vi "时间波形函数.vi"() -> ()   [LabVIEW 2023]
panel:
  out "Waveform Chart":waveform(dbl)[](graph)
  out "Waveform Graph 2":waveform(dbl)[](graph)
  out "appended array":waveform(dbl)[](array[waveform])
  out "Waveform Graph":waveform(dbl)(graph)
  out "output waveform":waveform(dbl)
  # "时间波形函数"
  # "t0（采样起始时间）、dt（采样间隔时间）、Y（数据，一维数组表示的每个点对应 Y 轴上的值）、attributes（波形的一些属性）"
  # "设置 和 读取 波形属性"
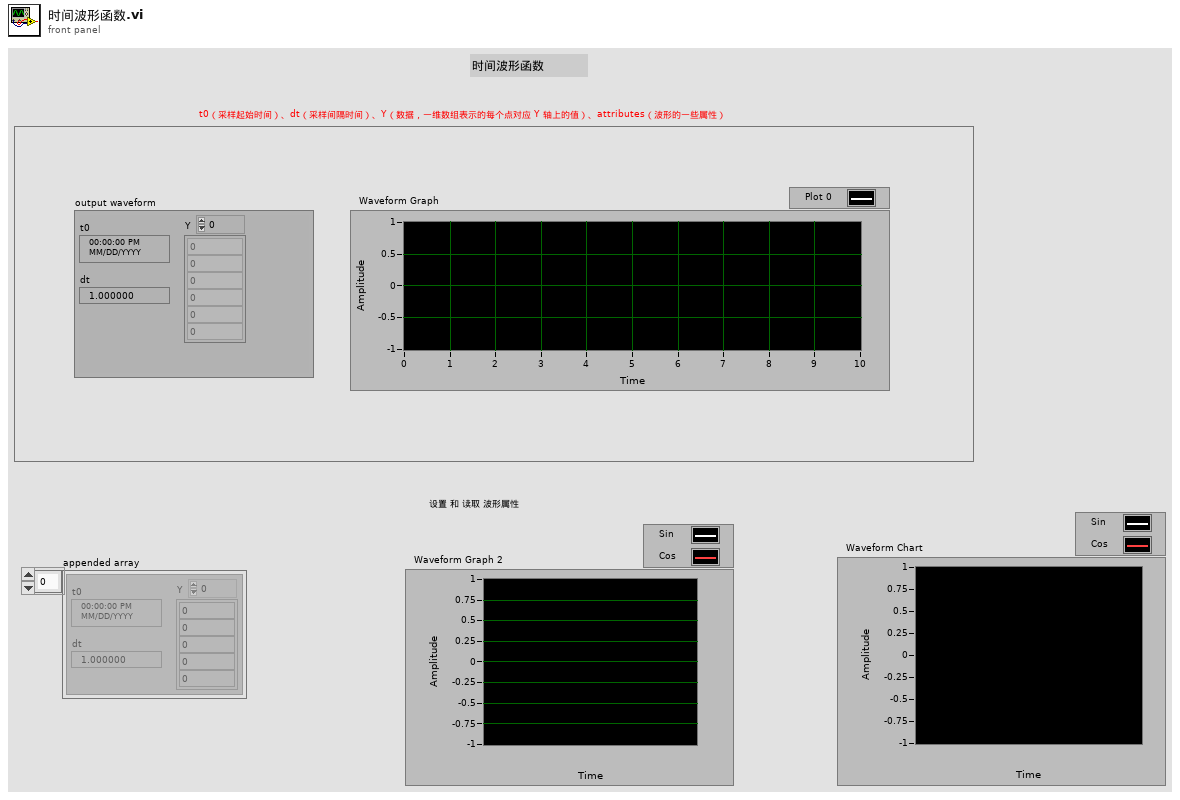
[diagram p1: front panel]
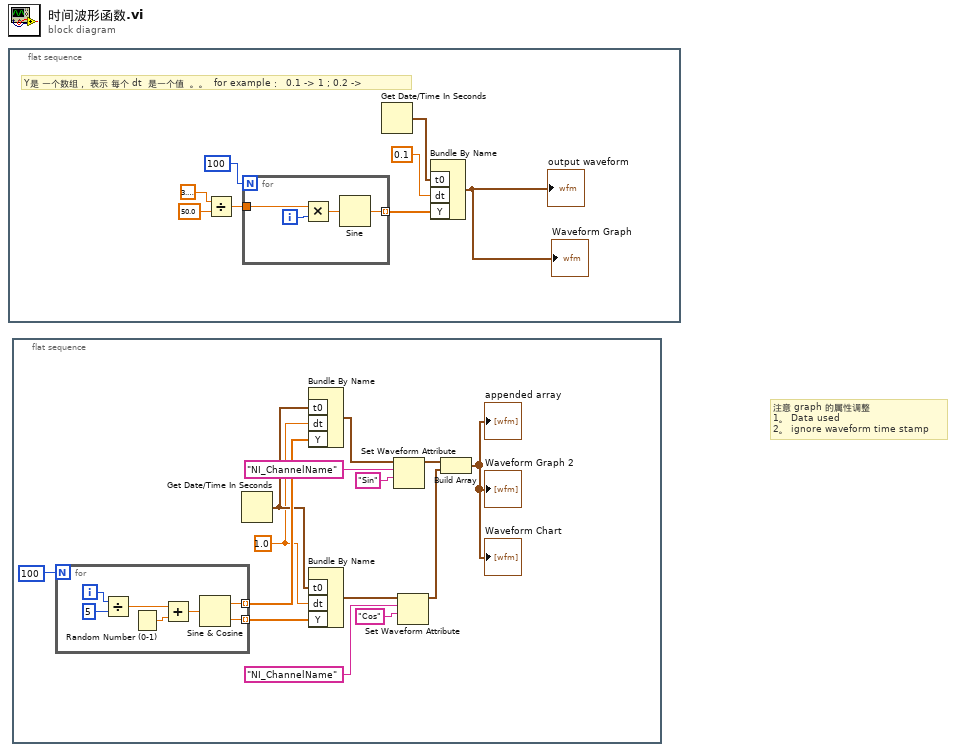
[diagram p0: block diagram]
diagram:
  # "注意 graph 的属性调整\n1。 Data used\n2。 ignore waveform time stamp"
  n1 = flat-sequence {
    frame #0 {
      # "Y是 一个数组， 表示 每个 dt  是一个值  。。  for example：  0.1 -> 1 ; 0.2 ->"
      n2 = Divide(x=3.141592653589793, y=50.0) -> (x/y=w5:dbl)
      n3 = for {
        N: 100 -> [_]
        tunnel: w5 -> [w12]
        tunnel: [w9] -> w2 mode=indexing
        i -> [w11]
        n4 = Multiply(x=w12, y=w11) -> (x*y=w10:dbl)
        n5 = Sine(x=w10) -> (sin(x)=w9:dbl)
      }
      n6 = Get Date/Time In Seconds() -> (seconds since 1Jan1904=w4:timestamp)
      n7 = Bundle By Name("t0"=w4, "dt"=0.1, "Y"=w2) -> (→"output waveform" →"Waveform Graph":waveform(dbl))  [unwired: 1 in]
    }
  }
  n8 = flat-sequence {
    frame #0 {
      w13 = 1.0 ("dt")
      n9 = for {
        N: 100 -> [_]
        tunnel: [w28] -> w25 mode=indexing
        tunnel: [w27] -> w24 mode=indexing
        i -> [w33]
        n10 = Divide(x=w33, y=5) -> (x/y=w31:dbl)
        n11 = Random Number (0-1)() -> (number: 0 to 1=w30:dbl)
        n12 = Add(x=w31, y=w30) -> (x+y=w29:dbl)
        n13 = Sine & Cosine(0:w29) -> (1:w28:dbl, 2:w27:dbl)
      }
      n14 = Get Date/Time In Seconds() -> (seconds since 1Jan1904=w23:timestamp)
      n15 = Bundle By Name("t0"=w23, "dt"=w13, "Y"=w25) -> (w22:waveform(dbl))  [unwired: 1 in]
      n16 = Bundle By Name("t0"=w23, "dt"=w13, "Y"=w24) -> (w19:waveform(dbl))  [unwired: 1 in]
      n17 = Set Waveform Attribute(5:"Sin", 6:"NI_ChannelName" ("name"), 7:w22) -> (3:w16:waveform(dbl))  [unwired: 1 in, 2 out]
      n18 = Set Waveform Attribute(5:"Cos", 6:"NI_ChannelName" ("name"), 7:w19) -> (3:w15:waveform(dbl))  [unwired: 1 in, 2 out]
      n19 = Build Array(w16, w15) -> (→"appended array" →"Waveform Graph 2" →"Waveform Chart":waveform(dbl)[])
    }
  }
